vi "Status Get Head Type.vi"(5 "Retry Attempts (0)":i32 min=0, 8 "error in":errorcluster, 11 "VISA resource name":refnum<visa-resource-name>) -> (0 "error out":errorcluster, 2 "Head Type":i32, 3 "VISA resource name out":refnum<visa-resource-name>)   [LabVIEW 2020, in "ChromTech Series III Pump.lvlib"]
doc: "Reads the pump head type, where:\n x = 1 for a stainless steel 10 mL/min pump head\n x = 2 for a plastic 10 mL/min pump head\n x = 3 for a stainless steel 40 mL/min pump head\n x = 4 for a plastic 40 mL/min pump head"
uses:
  ChromTech Series III Pump.lvlib
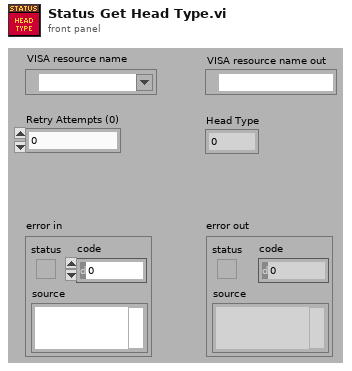
[diagram p1: front panel]
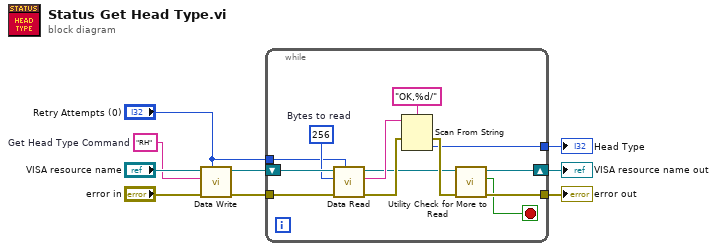
[diagram p0: block diagram]
diagram:
  w5 = "RH"  # Get Head Type Command
  n1 = call "Data Write.vi"("Retry Attempts (0)"="Retry Attempts (0)", "error in (no error)"="error in", "Command"=w5, "VISA Refnum in"="VISA resource name") -> ("error out"=w6:errorcluster, "VISA Refnum out"=w8:refnum<visa-resource-name>)  [unwired: 6 in]
  n2 = while {
    tunnel: [w17] -> w4
    shift-right: [w12] -> w2
    shift-left: w8 -> [w22]
    tunnel: "Retry Attempts (0)" -> [w10]
    tunnel: w6 -> [w21]
    tunnel: [w14] -> w3
    stop <- w11 stop-if-true
    w20 = u32 256  # Bytes to read
    n3 = call "Data Read.vi"("Retry Attempts (0)"=w10, "error in (no error)"=w21, "Bytes to read"=w20, "VISA Refnum in"=w22) -> ("error out"=w19:errorcluster, "read buffer"=w16:string, "VISA Refnum out"=w13:refnum<visa-resource-name>)  [unwired: 5 in]
    n4 = Scan From String(format string="OK,%d/", input string=w16, error in=w19) -> (error out=w18:errorcluster, output 1=w17:i32)  [unwired: 2 in, 2 out]
    n5 = call "Utility Check for More to Read.vi"("error in (no error)"=w18, "VISA Refnum in"=w13) -> ("error out (unchanged)"=w14:errorcluster, "More to read?"=w11:bool, "VISA Refnum out"=w12:refnum<visa-resource-name>)  [unwired: 7 in]
  }
  "VISA resource name out" <- w2
  "error out" <- w3
  "Head Type" <- w4
